vi "MountNAS.vi"(8 "error in":errorcluster) -> (0 "error out":errorcluster)   [LabVIEW 2018]
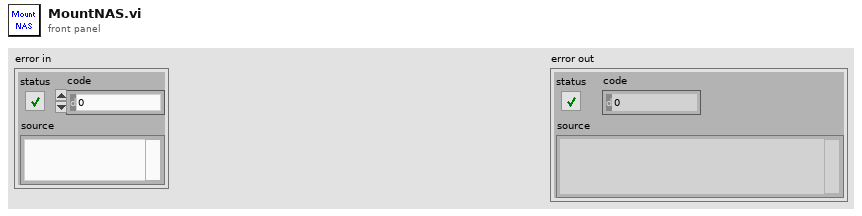
[diagram p1: front panel]
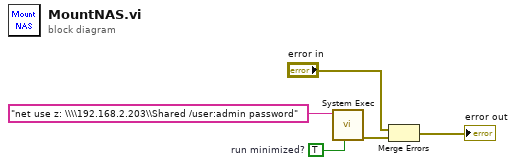
[diagram p0: block diagram]
diagram:
  w1 = TRUE  # run minimized?
  n1 = call <vilib>:"System Exec.vi"("run minimized? (F)"=w1, "command line"="net use z: \\\\192.168.2.203\\Shared /user:admin password" ("standard input")) -> ("error out"=w5:errorcluster)  [unwired: 6 in, 3 out]
  n2 = Merge Errors("error in", w5) -> (→"error out":errorcluster)
